vi "Create TCP Connection Handler.vi"(5 "TCPConnectionHandler in":refnum<class "TCPConnectionHandler.lvclass">, 8 "error in (no error)":errorcluster, 10 "NbConnections":refnum<user-event>, 11 "ServerRequest":refnum<queue>) -> (0 "error out":errorcluster, 3 "TCPConnectionHandler out":refnum<class "TCPConnectionHandler.lvclass">)   [LabVIEW 2013, in "MQTT Server.lvlib" / "TCPConnectionHandler.lvclass"]
uses:
  TCPConnectionHandler.lvclass
  MQTT_Base/Request -- cluster.ctl
  Control Packets/ControlPacket/ControlPacket.lvclass
  MQTT_Base/Response -- cluster.ctl
  TCPConnectionHandler.lvclass/TCPConnectionHandler.ctl
  process.vi
  MQTT_Base/MQTT_Base.lvclass
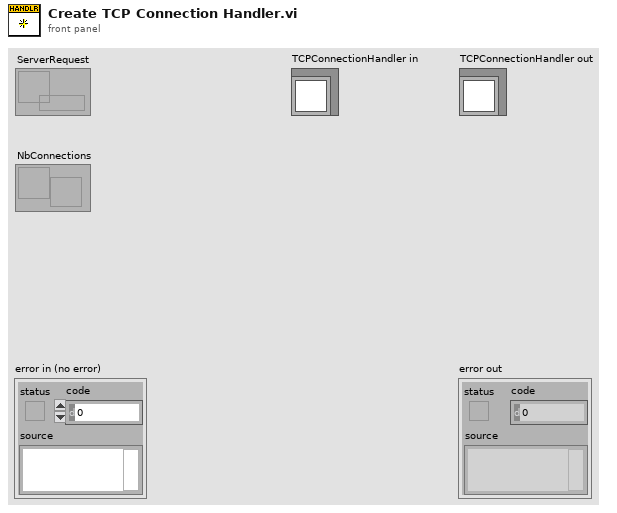
[diagram p1: front panel]
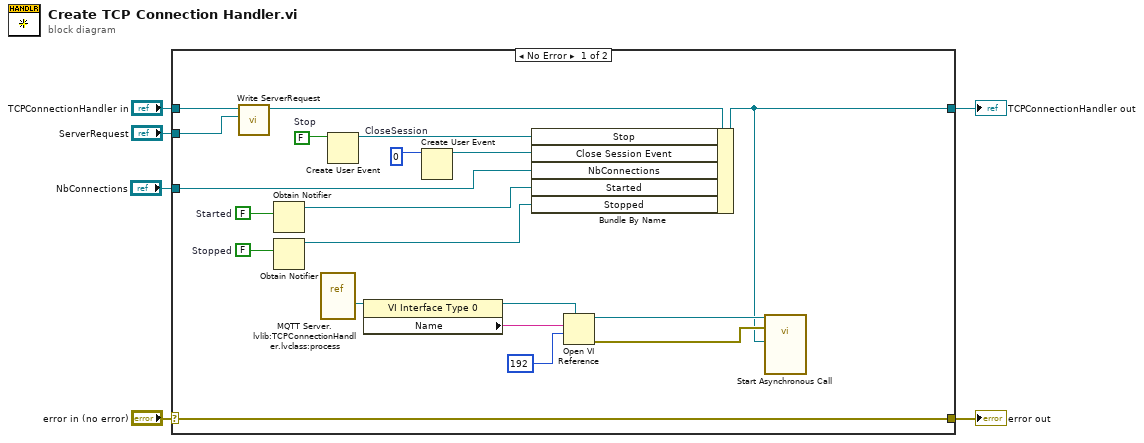
[diagram p0: block diagram]
diagram:
  n1 = case shown="No Error" "error in (no error)" {
    selector: "error in (no error)" -> [w26 w28]
    tunnel: [w26 w28] -> w5
    tunnel: [w14 w27] -> w3
    tunnel: "TCPConnectionHandler in" -> [w24 w27]
    tunnel: "ServerRequest" -> [w25 _]
    tunnel: "NbConnections" -> [w7 _]
    frame No Error {
      w10 = FALSE  # Stopped
      w11 = FALSE  # Started
      w13 = 0  # CloseSession
      w23 = FALSE  # Stop
      n2 = call "Write ServerRequest.vi"("ServerRequest"=w25, "TCPConnectionHandler in"=w24) -> ("TCPConnectionHandler out"=w21:refnum<class "TCPConnectionHandler.lvclass">)  [unwired: 9 in]
      n3 = Obtain Notifier(notification data type=w11) -> (notifier out=w9:refnum<notifier>)  [unwired: 3 in, 2 out]
      n4 = Obtain Notifier(notification data type=w10) -> (notifier out=w8:refnum<notifier>)  [unwired: 3 in, 2 out]
      n5 = vi-ref "MQTT Server.lvlib:TCPConnectionHandler.lvclass:process.vi"() -> (w20:refnum<vi>)
      n6 = Create User Event(user event datatype=w23) -> (user event=w22:refnum<user-event>)  [unwired: 1 in, 1 out]
      n7 = property class="VI Interface Type 0"(reference=w20) -> (reference out=w18:refnum<vi>, "Name"=w19:string)  [unwired: 1 in, 1 out]
      n8 = Create User Event(user event datatype=w13) -> (user event=w12:refnum<user-event>)  [unwired: 1 in, 1 out]
      n9 = Bundle By Name(cluster=w21, "Stop"=w22, "Close Session Event"=w12, "NbConnections"=w7, "Started"=w9, "Stopped"=w8) -> (w14:refnum<class "TCPConnectionHandler.lvclass">)
      n10 = Open VI Reference(type specifier VI Refnum (for type only)=w18, vi path=w19, options=192) -> (vi reference=w17:refnum<vi>, error out=w16:errorcluster)  [unwired: 3 in]
      n11 = call-by-ref "Start Asynchronous Call"(reference=w17, error in=w16, "TCPConnectionHandler in"=w14) -> ()  [unwired: 9 in, 4 out]
    }
    frame Error {
    }
  }
  "error out" <- w5
  "TCPConnectionHandler out" <- w3
